vi "Element Events.vi"(8 "error in (no error)":errorcluster, 11 "ImageButtonControl in":refnum<class "ImageButtonControl.lvclass">) -> (0 "error out":errorcluster, 2 "Element Events":refnum<class "Control Event Registrations.lvclass">, 3 "ImageButtonControl out":refnum<class "ImageButtonControl.lvclass">)   [LabVIEW 2020, in "VolatusGUIElements.lvlib" / "ImageButtonControl.lvclass"]
uses:
  ImageButtonControl.lvclass
  VolatusGUI/Control Event Registrations/Control Event Registrations.lvclass
  ImageButtonControl.lvclass/ImageButtonControl.ctl
  VolatusGUI/GUI Element/GUI Element.lvclass
  C:/dev/lv20CE/relink/lv-volatus/VolatusGUI/GUI Element/GUI Element.lvclass
  C:/dev/lv20CE/relink/lv-volatus/VolatusGUIElements/ImageButtonControl/ImageButtonControl.lvclass
  C:/dev/lv20CE/relink/lv-volatus/VolatusGUI/OnValueChangeHandler/OnValueChangeHandler.lvclass
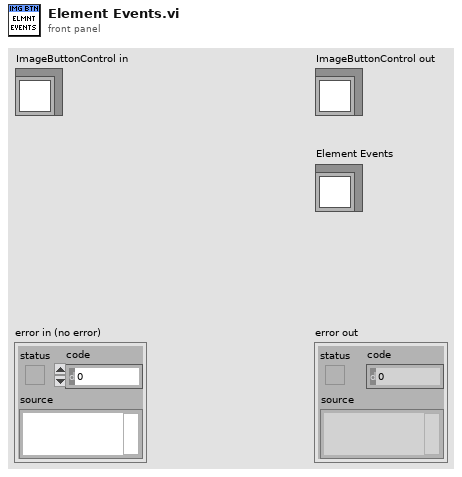
[diagram p1: front panel]
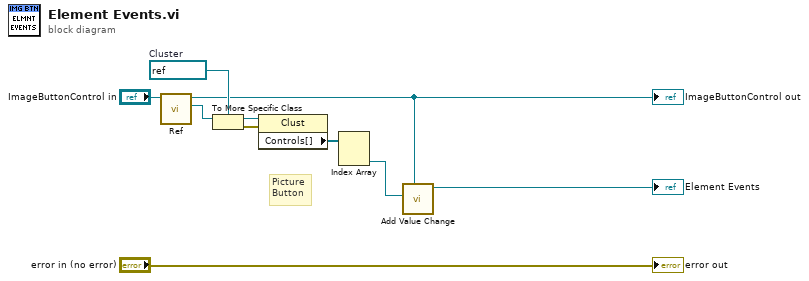
[diagram p0: block diagram]
diagram:
  w7 = refnum<vi> refnum  # Cluster
  # "Picture\nButton"
  n1 = call "Ref.vi"("GUI Element in"="ImageButtonControl in") -> ("Ref"=w8:refnum<vi>, "GUI Element out"=w2:refnum<class "ImageButtonControl.lvclass">)  [unwired: 9 in]
  "ImageButtonControl out" <- w2
  n2 = To More Specific Class(target class=w7, reference=w8) -> (specific class reference=w6:refnum<vi>, error out=w5:errorcluster)  [unwired: 1 in]
  n3 = property class="Clust"(reference=w6, error in=w5) -> ("Controls[]"=w4:refnum<vi>[])  [unwired: 2 out]
  n4 = Index Array(array=w4) -> (element #2=w1:refnum<vi>)  [unwired: 2 in, 1 out]
  n5 = call "Add Value Change.vi"("Control"=w2, "CtlRef"=w1) -> ("Control Event Registrations out"=→"Element Events":refnum<class "Control Event Registrations.lvclass">)  [unwired: 8 in, 1 out]
  "error out" <- "error in (no error)"
